vi "Prozentberechnung.vi"(8 "Grenzen Max":T1 {"Zahlen-Eingabefeld 16" format="%#_5g"; "Zahlen-Eingabefeld 15" format="%#_5g"; "Zahlen-Eingabefeld 14" format="%#_5g"; "Zahlen-Eingabefeld 13" format="%#_5g"; "Zahlen-Eingabefeld 12" format="%#_5g"; "Zahlen-Eingabefeld 11" format="%#_5g"; "Zahlen-Eingabefeld 10" format="%#_5g"; "Zahlen-Eingabefeld 9" format="%#_5g"; "Zahlen-Eingabefeld 8" format="%#_5g"; "Zahlen-Eingabefeld 7" format="%#_5g"; "Zahlen-Eingabefeld 6" format="%#_5g"; "Zahlen-Eingabefeld 5" format="%#_5g"; "Zahlen-Eingabefeld 4" format="%#_5g"; "Zahlen-Eingabefeld 3" format="%#_5g"; "Zahlen-Eingabefeld 2" format="%#_5g"; "Zahlen-Eingabefeld" format="%#_5g"}, 9 "Grenzen Min":T1 {"Zahlen-Eingabefeld 16" format="%#_5g"; "Zahlen-Eingabefeld 15" format="%#_5g"; "Zahlen-Eingabefeld 14" format="%#_5g"; "Zahlen-Eingabefeld 13" format="%#_5g"; "Zahlen-Eingabefeld 12" format="%#_5g"; "Zahlen-Eingabefeld 11" format="%#_5g"; "Zahlen-Eingabefeld 10" format="%#_5g"; "Zahlen-Eingabefeld 9" format="%#_5g"; "Zahlen-Eingabefeld 8" format="%#_5g"; "Zahlen-Eingabefeld 7" format="%#_5g"; "Zahlen-Eingabefeld 6" format="%#_5g"; "Zahlen-Eingabefeld 5" format="%#_5g"; "Zahlen-Eingabefeld 4" format="%#_5g"; "Zahlen-Eingabefeld 3" format="%#_5g"; "Zahlen-Eingabefeld 2" format="%#_5g"; "Zahlen-Eingabefeld" format="%#_5g"}, 11 "Aktuelle Werte":T3 {"Zahlen-Ausgabefeld 16" format="%#.2f"; "Zahlen-Ausgabefeld 15" format="%#.2f"; "Zahlen-Ausgabefeld 14" format="%#.2f"; "Zahlen-Ausgabefeld 13" format="%#.2f"; "Zahlen-Ausgabefeld 12" format="%#.2f"; "Zahlen-Ausgabefeld 11" format="%#.2f"; "Zahlen-Ausgabefeld 10" format="%#.2f"; "Zahlen-Ausgabefeld 9" format="%#.2f"; "Zahlen-Ausgabefeld 8" format="%#.2f"; "Zahlen-Ausgabefeld 7" format="%#.2f"; "Zahlen-Ausgabefeld 6" format="%#.2f"; "Zahlen-Ausgabefeld 5" format="%#.2f"; "Zahlen-Ausgabefeld 4" format="%#.2f"; "Zahlen-Ausgabefeld 3" format="%#.2f"; "Zahlen-Ausgabefeld 2" format="%#.2f"; "Zahlen-Ausgabefeld" format="%#.2f"}) -> (0 "Balken Anzeige":T4 {"Anzeige Balken 16" scale=0.0..100.0; "Anzeige Balken 15" scale=0.0..100.0; "Anzeige Balken 14" scale=0.0..100.0; "Anzeige Balken 13" scale=0.0..100.0; "Anzeige Balken 12" scale=0.0..100.0; "Anzeige Balken 11" scale=0.0..100.0; "Anzeige Balken 10" scale=0.0..100.0; "Anzeige Balken 9" scale=0.0..100.0; "Anzeige Balken 8" scale=0.0..100.0; "Anzeige Balken 7" scale=0.0..100.0; "Anzeige Balken 6" scale=0.0..100.0; "Anzeige Balken 5" scale=0.0..100.0; "Anzeige Balken 4" scale=0.0..100.0; "Anzeige Balken 3" scale=0.0..100.0; "Anzeige Balken 2" scale=0.0..100.0; "Anzeige Balken" scale=0.0..100.0})   [LabVIEW 2020, in "Gaszuordnung AO.lvlib"]
uses:
  Gaszuordnung AO.lvlib
  Balken Anzeige.ctl
  Balken.ctl
  Grenzen Anzeige.ctl
  Visualisierungs Elemente/Zahlen-Eingabefeld.ctl
  Aktuelle Werte Anzeige.ctl
  ANA-OUT Aktionen.ctl
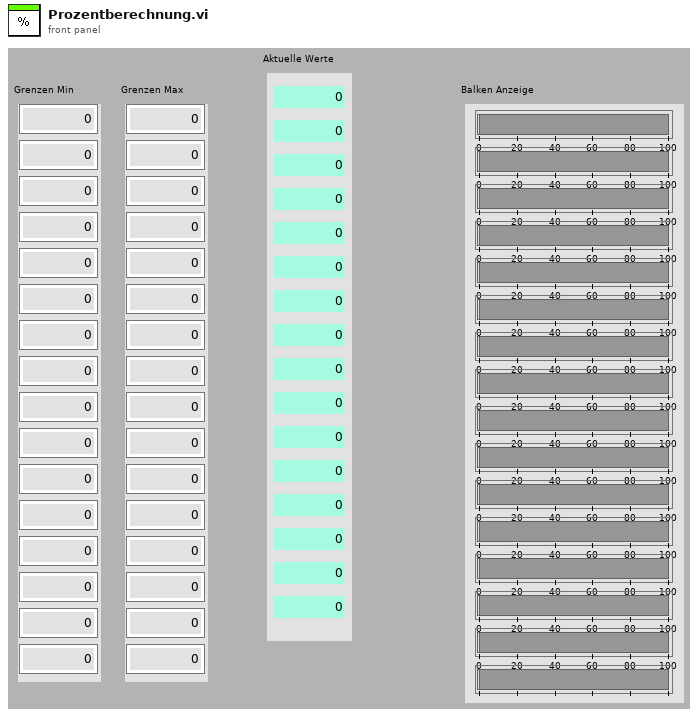
[diagram p1: front panel]
types:
  T1 = typedef "Gaszuordnung AO.lvlib/Grenzen Anzeige.ctl" = cluster{"Zahlen-Eingabefeld":T2, "Zahlen-Eingabefeld 2":T2, "Zahlen-Eingabefeld 3":T2, "Zahlen-Eingabefeld 4":T2, "Zahlen-Eingabefeld 5":T2, "Zahlen-Eingabefeld 6":T2, "Zahlen-Eingabefeld 7":T2, "Zahlen-Eingabefeld 8":T2, "Zahlen-Eingabefeld 9":T2, "Zahlen-Eingabefeld 10":T2, "Zahlen-Eingabefeld 11":T2, "Zahlen-Eingabefeld 12":T2, "Zahlen-Eingabefeld 13":T2, "Zahlen-Eingabefeld 14":T2, "Zahlen-Eingabefeld 15":T2, "Zahlen-Eingabefeld 16":T2}
  T2 = typedef "Zahlen-Eingabefeld.ctl" = sgl
  T3 = typedef "Gaszuordnung AO.lvlib/Aktuelle Werte Anzeige.ctl" = cluster{"Zahlen-Ausgabefeld":sgl, "Zahlen-Ausgabefeld 2":sgl, "Zahlen-Ausgabefeld 3":sgl, "Zahlen-Ausgabefeld 4":sgl, "Zahlen-Ausgabefeld 5":sgl, "Zahlen-Ausgabefeld 6":sgl, "Zahlen-Ausgabefeld 7":sgl, "Zahlen-Ausgabefeld 8":sgl, "Zahlen-Ausgabefeld 9":sgl, "Zahlen-Ausgabefeld 10":sgl, "Zahlen-Ausgabefeld 11":sgl, "Zahlen-Ausgabefeld 12":sgl, "Zahlen-Ausgabefeld 13":sgl, "Zahlen-Ausgabefeld 14":sgl, "Zahlen-Ausgabefeld 15":sgl, "Zahlen-Ausgabefeld 16":sgl}
  T4 = typedef "Gaszuordnung AO.lvlib/Balken Anzeige.ctl" = cluster{"Anzeige Balken":T5, "Anzeige Balken 2":T5, "Anzeige Balken 3":T5, "Anzeige Balken 4":T5, "Anzeige Balken 5":T5, "Anzeige Balken 6":T5, "Anzeige Balken 7":T5, "Anzeige Balken 8":T5, "Anzeige Balken 9":T5, "Anzeige Balken 10":T5, "Anzeige Balken 11":T5, "Anzeige Balken 12":T5, "Anzeige Balken 13":T5, "Anzeige Balken 14":T5, "Anzeige Balken 15":T5, "Anzeige Balken 16":T5}
  T5 = typedef "Gaszuordnung AO.lvlib/Balken.ctl" = u8
  T6 = typedef "Gaszuordnung AO.lvlib/ANA-OUT Aktionen.ctl" = enum16{"lesen", "Gase schreiben"}
  T7 = cluster{"[0]":T2, "[1]":T2, "[2]":T2, "[3]":T2, "[4]":T2, "[5]":T2, "[6]":T2, "[7]":T2, "[8]":T2, "[9]":T2, "[10]":T2, "[11]":T2, "[12]":T2, "[13]":T2, "[14]":T2, "[15]":T2}
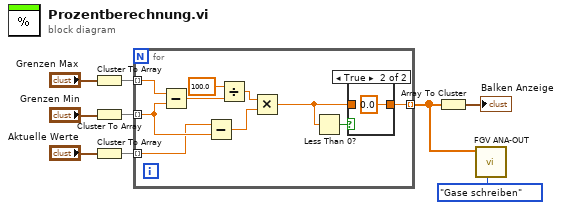
[diagram p0: block diagram]
diagram:
  n1 = Cluster To Array(cluster="Grenzen Max") -> (array=w4:T2[])
  n2 = Cluster To Array(cluster="Grenzen Min") -> (array=w5:T2[])
  n3 = Cluster To Array(cluster="Aktuelle Werte") -> (array=w7:sgl[])
  n4 = for {
    tunnel: w7 -> [w17] mode=indexing
    tunnel: w5 -> [w18] mode=indexing
    tunnel: w4 -> [w19] mode=indexing
    tunnel: [w12] -> w1 mode=indexing
    n5 = Subtract(x=w19, y=w18) -> (x-y=w16:T2)
    n6 = Subtract(x=w17, y=w18) -> (x-y=w14:T2)
    n7 = Divide(x=T2 100.0, y=w16) -> (x/y=w15:T2)
    n8 = Multiply(x=w15, y=w14) -> (x*y=w10:T2)
    n9 = Less Than 0?(x=w10) -> (x < 0?=w13:bool)
    n10 = case shown="True" w13 {
      tunnel: w10 -> [w20 _]
      tunnel: [w20 T2 0.0] -> w12
      frame False {
      }
      frame True {
      }
    }
  }
  n11 = Array To Cluster(array=w1) -> (cluster=→"Balken Anzeige":T7)
  n12 = call "FGV ANA-OUT.vi"("Aktion"=ANA-OUT_Aktionen."Gase schreiben", "ANA-OUT Gase"=w1) -> ()  [unwired: 9 in, 1 out]
